vi "Perform_large_file_Analysis.vi"(7 "error in":errorcluster) -> (2 "Wvfm":waveform(dbl)[](array[waveform]), 3 "Filtered Nb of Events":i32, 5 "Total Nb of Events":dbl)   [LabVIEW 2019]
uses:
  <vilib>/Utility/error.llb/DialogType.ctl
  ESA_Data_Analysis_Global_VIs.vi
  SiPM_Tests_Global_Var.vi
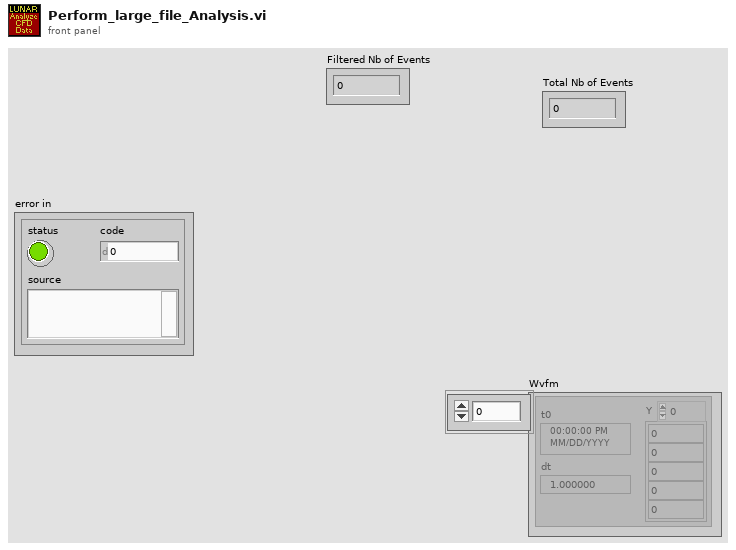
[diagram p1: front panel]
types:
  T1 = typedef "DialogType.ctl" = u16
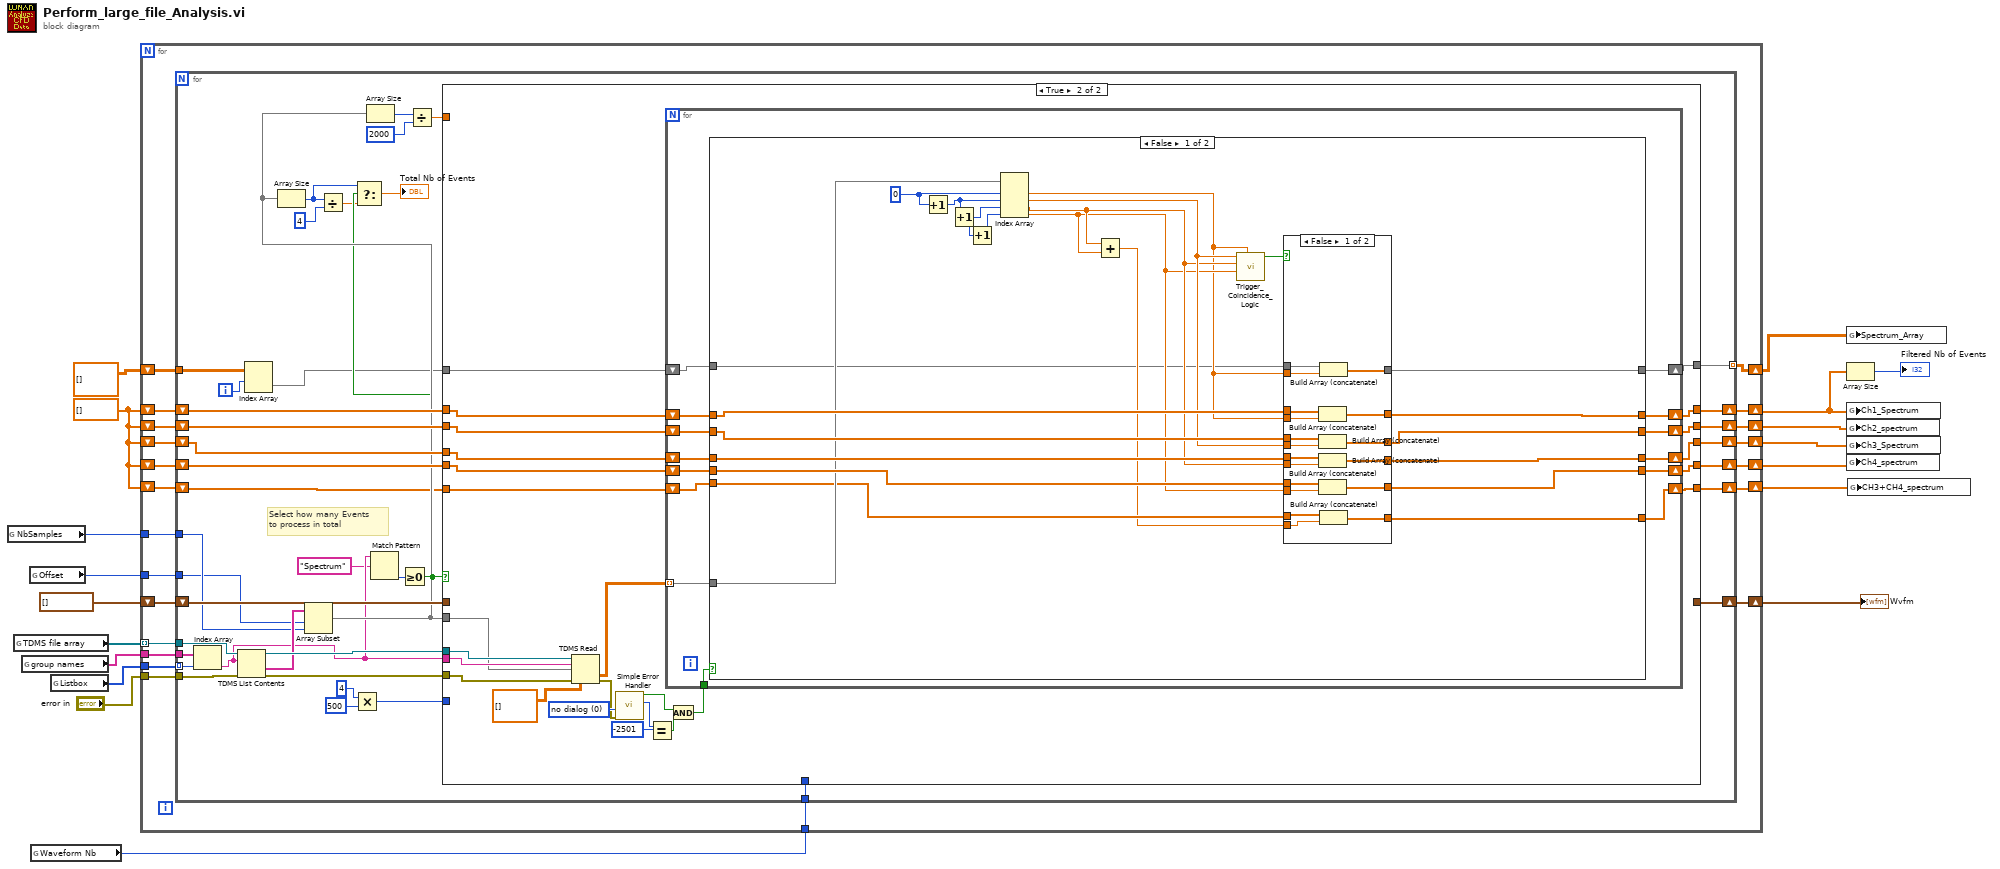
[diagram p0: block diagram]
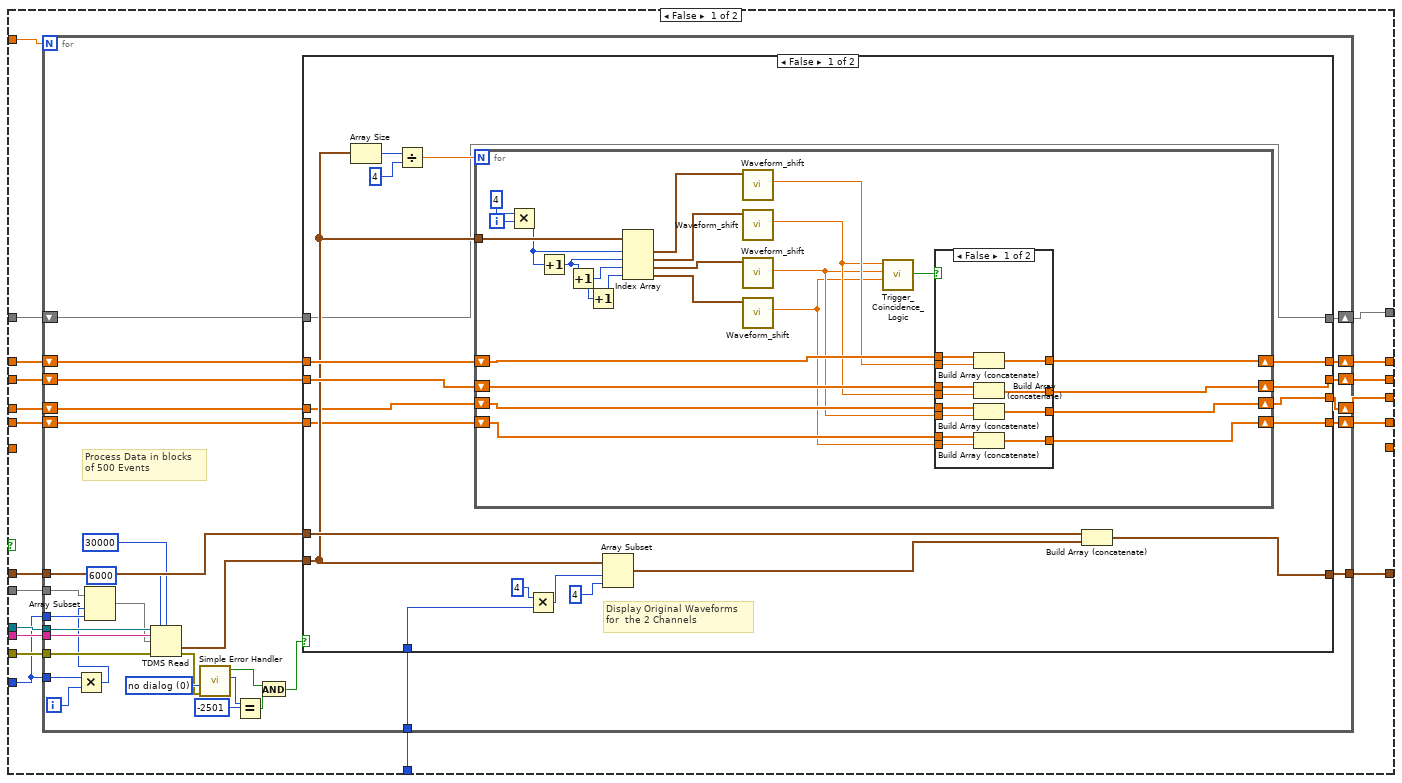
[diagram p2: hidden frame]
diagram:
  w5 = dbl[] []
  n1 = global read "SiPM_Tests_Global_Var.vi" "NbSamples"() -> (w12:i64)
  n2 = global read "SiPM_Tests_Global_Var.vi" "TDMS file array"() -> (w16:refnum<k34>[])
  n3 = global read "ESA_Data_Analysis_Global_VIs.vi" "group names"() -> (w18:string[])
  n4 = global read "SiPM_Tests_Global_Var.vi" "Offset"() -> (w14:i64)
  n5 = global read "SiPM_Tests_Global_Var.vi" "Waveform Nb"() -> (w11:u16)
  n6 = global read "ESA_Data_Analysis_Global_VIs.vi" "Listbox"() -> (w1:i32[])
  n7 = for {
    tunnel: w16 -> [w39] mode=indexing
    tunnel: w18 -> [w38]
    tunnel: w1 -> [w37]
    tunnel: "error in" -> [w36]
    tunnel: w14 -> [w34]
    shift-right: [w35] -> w15
    shift-left: waveform(dbl)[] [] -> [w33]
    shift-right: [w29] -> w10
    shift-left: w5 -> [w32]
    shift-right: [w30] -> w7
    shift-left: w5 -> [w31]
    tunnel: w12 -> [w28]
    tunnel: w11 -> [w27]
    shift-right: [w24] -> w9
    shift-left: w5 -> [w26]
    shift-right: [w23] -> w8
    shift-left: w5 -> [w25]
    shift-right: [w21] -> w4
    shift-left: w5 -> [w22]
    shift-right: [w19] -> w2
    shift-left: dbl[][] [] -> [w20]
    n8 = for {
      tunnel: w39 -> [w80]
      tunnel: w38 -> [w79]
      tunnel: w37 -> [w78] mode=indexing
      tunnel: w36 -> [w77]
      tunnel: w34 -> [w40]
      shift-right: [w74] -> w35
      shift-left: w33 -> [w73]
      shift-right: [w70] -> w29
      shift-left: w32 -> [w72]
      shift-right: [w46] -> w30
      shift-left: w31 -> [w71]
      tunnel: w28 -> [w41]
      tunnel: w27 -> [w69]
      shift-right: [w66] -> w24
      shift-left: w26 -> [w68]
      shift-right: [w65] -> w23
      shift-left: w25 -> [w67]
      shift-right: [w47] -> w21
      shift-left: w22 -> [w48]
      tunnel: [w45] -> w19 mode=indexing
      tunnel: w20 -> [w44]
      i -> [w43]
      # "Select how many Events \nto process in total"
      n9 = Index Array(array=w79, index=w78) -> (element=w55:string)
      n10 = TDMS List Contents(4:w77, 6:w55, 7:w80) -> (0:w75:errorcluster, 1:w64:string[], 3:w76:refnum<k34>)  [unwired: 1 out]
      n11 = Index Array(array=w44, index (row)=w43) -> (element=w42:dbl[])  [unwired: 1 in]
      n12 = Array Subset(array=w64, index=w40, length=w41) -> (w56:string[])
      n13 = Array Size(array=w56) -> (size(s)=w51:i32)
      n14 = Divide(x=w51, y=4) -> (x/y=w50:dbl)
      n15 = Multiply(x=i64 4, y=i64 500) -> (x*y=w61:i64)
      n16 = Array Size(array=w56) -> (size(s)=w59:i32)
      n17 = Match Pattern(string=w55, regular expression="Spectrum") -> (offset past match=w53:i32)  [unwired: 1 in, 3 out]
      n18 = Greater Or Equal To 0?(x=w53) -> (x >= 0?=w52:bool)
      n19 = Select(t=w51, s=w52, f=w50) -> (s? t:f=→"Total Nb of Events":dbl)
      n20 = Divide(x=w59, y=2000) -> (x/y=w58:dbl)
      n21 = case shown="True" w52 {
        tunnel: w76 -> [w99 w220]
        tunnel: w55 -> [w98 w221]
        tunnel: w75 -> [w97 w222]
        tunnel: [w96 _] -> w74
        tunnel: w73 -> [w95 _]
        tunnel: w72 -> [w94 w210]
        tunnel: w71 -> [w93 w211]
        tunnel: [w92 w207] -> w46
        tunnel: [w91 w206] -> w70
        tunnel: w69 -> [w90 _]
        tunnel: w68 -> [w89 w209]
        tunnel: w67 -> [w88 w208]
        tunnel: [w87 w205] -> w66
        tunnel: [w86 w204] -> w65
        tunnel: w61 -> [w85 _]
        tunnel: w58 -> [w84 _]
        tunnel: w56 -> [w83 w203]
        tunnel: w48 -> [_ w201]
        tunnel: [_ w200] -> w47
        tunnel: [w81 w199] -> w45
        tunnel: w42 -> [w82 w198]
        frame False {
          n22 = for {
            N: w84 -> [_]
            tunnel: w99 -> [w131]
            tunnel: w98 -> [w130]
            tunnel: w97 -> [w127]
            tunnel: [w126] -> w96
            tunnel: w95 -> [w125]
            tunnel: w90 -> [w115]
            tunnel: w83 -> [w109]
            shift-right: [w117] -> w92
            shift-left: w93 -> [w118]
            shift-right: [w116] -> w91
            shift-left: w94 -> [w119]
            shift-right: [w112] -> w87
            shift-left: w89 -> [w114]
            shift-right: [w111] -> w86
            shift-left: w88 -> [w113]
            tunnel: w85 -> [w107]
            tunnel: w85 -> [w105]
            shift-right: [w101] -> w81
            shift-left: w82 -> [w100]
            i -> [w106]
            w129 = T1 0 items=["no dialog", "OK message", "continue or stop message", "OK message + warnings", "continue/stop + warnings"] ("type of dialog (OK msg:1)")
            # "Process Data in blocks \nof 500 Events"
            n23 = Multiply(x=w105, y=w106) -> (x*y=w104:i64)
            n24 = Array Subset(array=w109, index=w104, length=w107) -> (w108:string[])
            n25 = TDMS Read(0:w131, 1:i64 6000 ("offset (0)"), 2:i64 30000 ("count (-1: all)"), 5:w130, 7:w108, 11:w127) -> (10:w110:waveform(dbl)[], 15:w128:errorcluster)  [unwired: 2 in, 4 out]
            n26 = call <vilib>:"Simple Error Handler.vi"("type of dialog (OK msg:1)"=w129, "error in (no error)"=w128) -> ("error?"=w123:bool, "code out"=w122:i32)  [unwired: 3 in, 3 out]
            n27 = Equal?(x=w122, y=-2501) -> (x = y?=w120:bool)
            n28 = And(x=w123, y=w120) -> (x .and. y?=w124:bool)
            n29 = case shown="False" w124 {
              tunnel: w110 -> [w137 _]
              tunnel: [w150 w197] -> w126
              tunnel: w125 -> [w149 w197]
              tunnel: w119 -> [w145 w195]
              tunnel: w118 -> [w144 w196]
              tunnel: [w143 w196] -> w117
              tunnel: [w142 w195] -> w116
              tunnel: w115 -> [w138 _]
              tunnel: w114 -> [w136 w194]
              tunnel: w113 -> [w135 w193]
              tunnel: [w134 w194] -> w112
              tunnel: [w133 w193] -> w111
              tunnel: [w132 w192] -> w101
              tunnel: w100 -> [w132 w192]
              frame False {
                # "Display Original Waveforms\nfor  the 2 Channels"
                n30 = Array Size(array=w137) -> (size(s)=w148:i32)
                n31 = Divide(x=w148, y=4) -> (x/y=w146:dbl)
                n32 = for {
                  N: w146 -> [_]
                  tunnel: w137 -> [w175]
                  shift-right: [w162] -> w143
                  shift-left: w144 -> [w163]
                  shift-right: [w160] -> w142
                  shift-left: w145 -> [w170]
                  shift-right: [w158] -> w134
                  shift-left: w136 -> [w159]
                  shift-right: [w157] -> w133
                  shift-left: w135 -> [w156]
                  i -> [w169]
                  n33 = Multiply(x=4, y=w169) -> (x*y=w173:i32)
                  n34 = Increment(x=w173) -> (x+1=w168:i32)
                  n35 = Increment(x=w168) -> (x+1=w166:i32)
                  n36 = Increment(x=w166) -> (x+1=w167:i32)
                  n37 = Index Array(array=w175, index #1=w173, index #2=w168, index #3=w166, index #4=w167) -> (element #1=w172:waveform(dbl), element #2=w171:waveform(dbl), element #3=w165:waveform(dbl), element #4=w164:waveform(dbl))
                  n38 = call "Waveform_shift.vi"("Waveform_in"=w172) -> ("Peak Value"=w161:dbl)  [unwired: 9 in]
                  n39 = call "Waveform_shift.vi"("Waveform_in"=w171) -> ("Peak Value"=w154:dbl)  [unwired: 9 in]
                  n40 = call "Waveform_shift.vi"("Waveform_in"=w165) -> ("Peak Value"=w153:dbl)  [unwired: 9 in]
                  n41 = call "Waveform_shift.vi"("Waveform_in"=w164) -> ("Peak Value"=w152:dbl)  [unwired: 9 in]
                  n42 = call "Trigger_Coincidence_Logic.vi"("Peak_ch4"=w152, "Peak_ch3"=w153, "Peak_ch2"=w154) -> ("Filter-out"=w155:bool)  [unwired: 8 in]
                  n43 = case shown="False" w155 {
                    tunnel: w170 -> [w187 w190]
                    tunnel: w154 -> [w186 _]
                    tunnel: w163 -> [w185 w191]
                    tunnel: [w184 w191] -> w162
                    tunnel: w161 -> [w183 _]
                    tunnel: [w182 w190] -> w160
                    tunnel: w159 -> [w181 w189]
                    tunnel: w153 -> [w180 _]
                    tunnel: [w179 w189] -> w158
                    tunnel: [w178 w188] -> w157
                    tunnel: w156 -> [w177 w188]
                    tunnel: w152 -> [w176 _]
                    frame False {
                      n44 = Build Array (concatenate)(w185, w183) -> (w184:dbl[])
                      n45 = Build Array (concatenate)(w187, w186) -> (w182:dbl[])
                      n46 = Build Array (concatenate)(w181, w180) -> (w179:dbl[])
                      n47 = Build Array (concatenate)(w177, w176) -> (w178:dbl[])
                    }
                    frame True {
                    }
                  }
                }
                n48 = Multiply(x=4, y=w138) -> (x*y=w141:i32)
                n49 = Array Subset(array=w137, index=w141, length=4) -> (w151:waveform(dbl)[])
                n50 = Build Array (concatenate)(w149, w151) -> (w150:waveform(dbl)[])
              }
              frame True {
              }
            }
          }
        }
        frame True {
          w219 = T1 0 items=["no dialog", "OK message", "continue or stop message", "OK message + warnings", "continue/stop + warnings"] ("type of dialog (OK msg:1)")
          n51 = TDMS Read(0:w220, 5:w221, 7:w203, 11:w222, 12:dbl[][] []) -> (10:w212:dbl[][], 15:w218:errorcluster)  [unwired: 3 in, 4 out]
          n52 = call <vilib>:"Simple Error Handler.vi"("type of dialog (OK msg:1)"=w219, "error in (no error)"=w218) -> ("error?"=w216:bool, "code out"=w215:i32)  [unwired: 3 in, 3 out]
          n53 = Equal?(x=w215, y=-2501) -> (x = y?=w213:bool)
          n54 = And(x=w216, y=w213) -> (x .and. y?=w217:bool)
          n55 = for {
            tunnel: w217 -> [w236]
            tunnel: w212 -> [w235] mode=indexing
            shift-right: [w227] -> w204
            shift-left: w208 -> [w231]
            shift-right: [w228] -> w205
            shift-left: w209 -> [w232]
            shift-right: [w229] -> w206
            shift-left: w210 -> [w233]
            shift-right: [w230] -> w207
            shift-left: w211 -> [w234]
            shift-right: [w225] -> w200
            shift-left: w201 -> [w226]
            shift-right: [w224] -> w199
            shift-left: w198 -> [w223]
            n56 = case shown="False" w236 {
              tunnel: w233 -> [w259 w288]
              tunnel: w234 -> [w258 w289]
              tunnel: [w257 w289] -> w230
              tunnel: [w256 w288] -> w229
              tunnel: w232 -> [w255 w287]
              tunnel: w231 -> [w254 w286]
              tunnel: [w253 w287] -> w228
              tunnel: [w252 w286] -> w227
              tunnel: w235 -> [w251 _]
              tunnel: w226 -> [w242 w285]
              tunnel: [w240 w285] -> w225
              tunnel: [w239 w284] -> w224
              tunnel: w223 -> [w237 w284]
              frame False {
                w245 = 0 ("x")
                n57 = Increment(x=w245) -> (x+1=w250:i32)
                n58 = Increment(x=w250) -> (x+1=w248:i32)
                n59 = Increment(x=w248) -> (x+1=w249:i32)
                n60 = Index Array(array=w251, index #1=w245, index #2=w250, index #3=w248, index #4=w249) -> (element #1=w238:dbl, element #2=w246:dbl, element #3=w244:dbl, element #4=w243:dbl)
                n61 = Add(x=w244, y=w243) -> (x+y=w241:dbl)
                n62 = call "Trigger_Coincidence_Logic.vi"("Peak_ch1"=w238, "Peak_ch4"=w243, "Peak_ch3"=w244, "Peak_ch2"=w246) -> ("Filter-out"=w247:bool)  [unwired: 7 in]
                n63 = case shown="False" w247 {
                  tunnel: w259 -> [w277 w282]
                  tunnel: w246 -> [w276 _]
                  tunnel: w258 -> [w275 w283]
                  tunnel: [w274 w283] -> w257
                  tunnel: w238 -> [w273 _]
                  tunnel: [w272 w282] -> w256
                  tunnel: w255 -> [w271 w281]
                  tunnel: w244 -> [w270 _]
                  tunnel: [w269 w281] -> w253
                  tunnel: [w268 w280] -> w252
                  tunnel: w254 -> [w267 w280]
                  tunnel: w243 -> [w266 _]
                  tunnel: w242 -> [w265 w279]
                  tunnel: w241 -> [w264 _]
                  tunnel: [w263 w279] -> w240
                  tunnel: [w262 w278] -> w239
                  tunnel: w238 -> [w261 _]
                  tunnel: w237 -> [w260 w278]
                  frame False {
                    n64 = Build Array (concatenate)(w275, w273) -> (w274:dbl[])
                    n65 = Build Array (concatenate)(w277, w276) -> (w272:dbl[])
                    n66 = Build Array (concatenate)(w271, w270) -> (w269:dbl[])
                    n67 = Build Array (concatenate)(w267, w266) -> (w268:dbl[])
                    n68 = Build Array (concatenate)(w260, w261) -> (w262:dbl[])
                    n69 = Build Array (concatenate)(w265, w264) -> (w263:dbl[])
                  }
                  frame True {
                  }
                }
              }
              frame True {
              }
            }
          }
        }
      }
    }
  }
  "Wvfm" <- w15
  n70 = global write "SiPM_Tests_Global_Var.vi" "Spectrum_Array"(w2) -> ()
  n71 = Array Size(array=w7) -> (size(s)=→"Filtered Nb of Events":i32)
  n72 = global write "SiPM_Tests_Global_Var.vi" "Ch1_Spectrum"(w7) -> ()
  n73 = global write "SiPM_Tests_Global_Var.vi" "Ch2_spectrum"(w10) -> ()
  n74 = global write "SiPM_Tests_Global_Var.vi" "Ch3_Spectrum"(w9) -> ()
  n75 = global write "SiPM_Tests_Global_Var.vi" "Ch4_spectrum"(w8) -> ()
  n76 = global write "SiPM_Tests_Global_Var.vi" "CH3+CH4_spectrum"(w4) -> ()
